vi "Check for Event.vi"(8 "error in (no error)":errorcluster, 11 "Muon Detector in":refnum<class "Muon Detector.lvclass">) -> (0 "error out":errorcluster, 1 "Valid?":bool, 2 "Event":T1, 3 "Muon Detector out":refnum<class "Muon Detector.lvclass">)   [LabVIEW 2019, in "Muon Detector.lvclass"]
uses:
  Muon Detector.lvclass
  Event.ctl
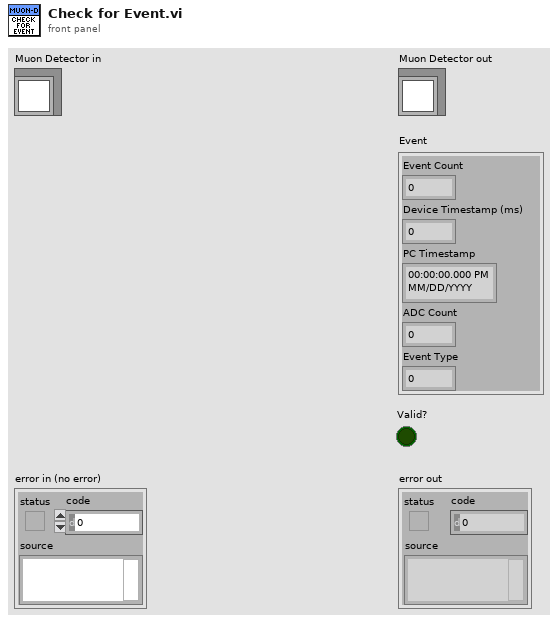
[diagram p1: front panel]
types:
  T1 = typedef "Muon Detector.lvclass/Event.ctl" = cluster{"Event Count":i32, "Device Timestamp (ms)":i32, "PC Timestamp":timestamp, "ADC Count":i32, "Event Type":u8}
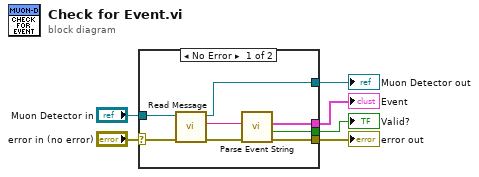
[diagram p0: block diagram]
diagram:
  n1 = case shown="No Error" "error in (no error)" {
    selector: "error in (no error)" -> [w14 w16]
    tunnel: [w9 w16] -> w5
    tunnel: [w12 w15] -> w3
    tunnel: "Muon Detector in" -> [w13 w15]
    tunnel: [w8 _] -> w2
    tunnel: [w7 _] -> w1
    frame No Error {
      n2 = call-dynamic "Read Message.vi"("error in (no error)"=w14, "Muon Detector in"=w13) -> ("error out"=w10:errorcluster, "Message"=w11:string, "Muon Detector out"=w12:refnum<class "Muon Detector.lvclass">)  [unwired: 7 in]
      n3 = call "Parse Event String.vi"("error in (no error)"=w10, "Message"=w11) -> ("error out"=w9:errorcluster, "Valid?"=w7:bool, "Event"=w8:T1)  [unwired: 7 in]
    }
    frame Error {
    }
  }
  "error out" <- w5
  "Muon Detector out" <- w3
  "Event" <- w2
  "Valid?" <- w1
